vi "read (in place).vi"(8 "error in (no error)":errorcluster, 10 "preallocated data in":string, 11 "file descriptor in":i32) -> (0 "error out":errorcluster, 1 "bytes read":i32, 2 "data out":string, 3 "file descriptor out":i32)   [LabVIEW 2016, in "Linux RT IPC.C.lvlib"]
uses:
  Linux RT IPC.C.lvlib
  Controls/functions.ctl
  <vilib>/NI/NI Linux RT Errno/Linux Errno.lvlib
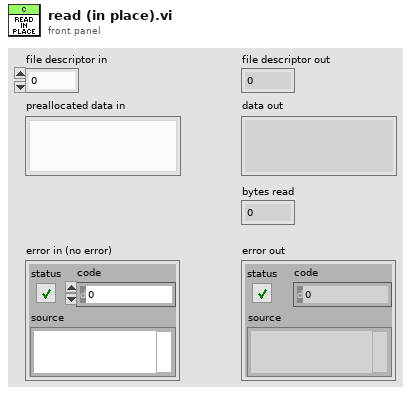
[diagram p1: front panel]
types:
  T1 = typedef "Linux RT IPC.C.lvlib/functions.ctl" = enum16{"unspecified", "close", "epoll_create", "epoll_ctl", "epoll_wait", "fstat", "ftruncate", "mkfifo", "mmap", "munmap", "open", "read", "shm_open", "shm_unlink", "timerfd_create", "timerfd_settime", "timerfd_gettime", "write", "unlink"}
  T2 = typedef "Linux Errno.lvlib/errno.ctl" = enum16{"NO ERROR", "EPERM", "ENOENT", "ESRCH", "EINTR", "EIO", "ENXIO", "E2BIG", "ENOEXEC", "EBADF", "ECHILD", "EAGAIN", "ENOMEM", "EACCES", "EFAULT", "ENOTBLK", "EBUSY", "EEXIST", "EXDEV", "ENODEV", "ENOTDIR", "EISDIR", "EINVAL", "ENFILE", "EMFILE", "ENOTTY", "ETXTBSY", "EFBIG", "ENOSPC", "ESPIPE", "EROFS", "EMLINK", "EPIPE", "EDOM", "ERANGE", "EDADLK", "ENAMETOOLONG", "ENOLCK", "ENOSYS", "ENOTEMPTY", "ELOOP", "EWOULDBLOCK", "ENOMSG", "EIDRM", "ECHRNG", "EL2NSYNC", "EL3HLT", "EL3RST", "ELNRNG", "EUNATCH", "ENOCSI", "EL2HLT", "EBADE", "EBADR", "EXFULL", "ENOANO", "EBADRQC", "EBADSLT", "EDEADLOCK", "EBFONT", "ENOSTR", "ENODATA", "ETIME", "ENOSR", "ENONET", "ENOPKG", "EREMOTE", "ENOLINK", "EADV", "ESRMNT", "ECOMM", "EPROTO", "EMULTIHOP", "EDOTDOT", "EBADMSG", "EOVERFLOW", "ENOTUNIQ", "EBADFD", "EREMCHG", "ELIBACC", "ELIBBAD", "ELIBSCN", "ELIBMAX", "ELIBEXEC", "ELISEQ", "ERESTART", "ESTRPIPE", "EUSERS", "ENOTSOCK", "EDESTADDRREQ", "EMSGSIZE", "EPROTOTYPE", "ENOPROTOOPT", "EPROTONOSUPPORT", "ESOCKTNOSUPPORT", "EOPNOTSUPP", "EPFNOSUPPORT", "EAFNOSUPPORT", "EADDRINUSE", "EADDRNOTAVAIL", "ENETDOWN", "ENETUNREACH", "ENETRESET", "ECONNABORTED", "ECONNRESET", "ENOBUFS", "EISCONN", "ENOTCONN", "ESHUTDOWN", "ETOOMANYREFS", "ETIMEDOUT", "ECONNREFUSED", "EHOSTDOWN", "EHOSTUNREACH", "EALREADY", "EINPROGRESS", "ESTALE", "EUCLEAN", "ENOTNAM", "ENAVAIL", "EISNAM", "EREMOTEIO", "EDQUOT", "ENOMEDIUM", "EMEDIUMTYPE", "ECANCELED", "ENOKEY", "EKEYEXPIRED", "EKEYREVOKED", "EKEYREJECTED", "EOWNERDEAD", "ENOTRECOVERABLE", "ERFKILL", "EHWPOISON", "UNDEFINED"}
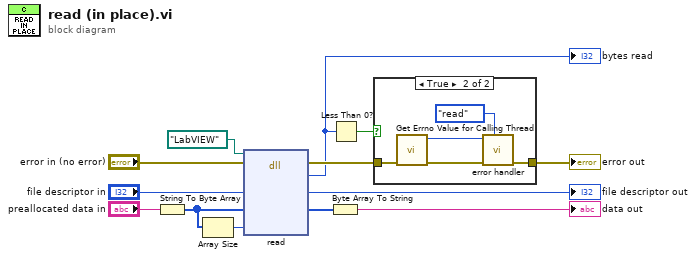
[diagram p0: block diagram]
diagram:
  n1 = String To Byte Array(string="preallocated data in") -> (unsigned byte array=w1:u8[])
  n2 = Array Size(array=w1) -> (size(s)=w2:i32)
  n3 = dll-call lib="LabVIEW" fn="read"(path in=path "LabVIEW", error in="error in (no error)", "fd"="file descriptor in", "buf"=w1, "count"=w2) -> (error out=w9:errorcluster, "return"=w6:i32, "fd"=→"file descriptor out":i32, "buf"=w11:u8[])  [unwired: 2 in, 1 out]
  "bytes read" <- w6
  n4 = Byte Array To String(unsigned byte array=w11) -> (string=→"data out":string)
  n5 = Less Than 0?(x=w6) -> (x < 0?=w8:bool)
  n6 = case shown="True" w8 {
    tunnel: w9 -> [w14 w19]
    tunnel: [w14 w18] -> w7
    frame False {
    }
    frame True {
      n7 = call <vilib>:"Get Errno Value for Calling Thread.vi"("error in (no error)"=w19) -> ("error out"=w16:errorcluster, "errno"=w17:T2)  [unwired: 9 in]
      n8 = call "error handler.vi"("function (unspecified)"=functions."read" ("function"), "error in (no error)"=w16, "errno"=w17) -> ("error out"=w18:errorcluster)  [unwired: 8 in]
    }
  }
  "error out" <- w7
